vi "Actor Core.vi"(8 "error in":errorcluster, 11 "Jobber Proxy in":refnum<class "Jobber Proxy.lvclass">) -> (0 "error out":errorcluster, 3 "Actor out":refnum<class "Actor.lvclass">)   [LabVIEW 2014, in "Jobber Proxy.lvlib" / "Jobber Proxy.lvclass"]
doc: "(<B>Filename</B>: Actor Framework.lvlib:Actor.lvclass:Actor Core.vi)\n\nReceives messages to the actor, reacts to them, and initiates any error handling that may shut the actor down.\n\nDescendant classes may override this VI to append parallel tasks for the actor to complete while it handles messages. Overrides use the Call Parent Method node."
uses:
  Jobber Proxy.lvclass
  <vilib>/ActorFramework/Actor/Actor.lvclass
  Jobber/Jobber/Jobber.lvclass
  Jobber Proxy.lvclass/Jobber Proxy.ctl
  Jobber/Jobber/Jobber.lvclass/Jobber.ctl
  Classes/LabVIEW Instance/LabVIEW Instance.lvclass
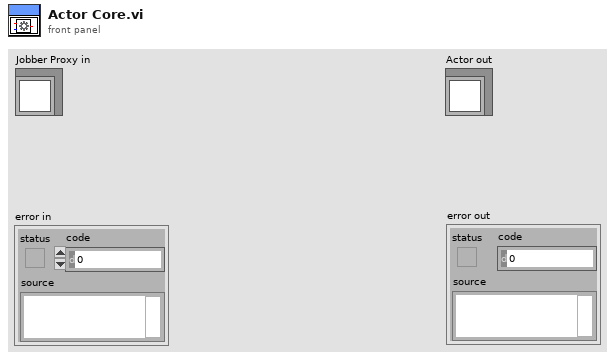
[diagram p1: front panel]
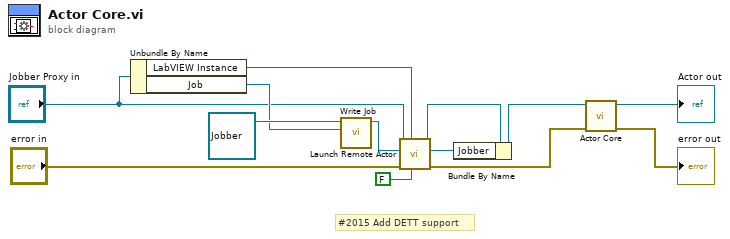
[diagram p0: block diagram]
diagram:
  # "#2015 Add DETT support"
  n1 = Unbundle By Name("Jobber Proxy in") -> ("LabVIEW Instance"=w6:refnum<class "LabVIEW Instance.lvclass">, "Job"=w7:refnum<class "Job.lvclass">)
  n2 = call "Write Job.vi"("Job.lvclass"=w7, "Jobber in"=refnum<class "Jobber.lvclass"> refnum ("Jobber.lvlib:Jobber.lvclass")) -> ("Jobber out"=w5:refnum<class "Jobber.lvclass">)  [unwired: 9 in]
  n3 = call "Launch Remote Actor.vi"("Open Actor Core front panel? (F)"=FALSE, "LabVIEW Instance in"=w6, "error in (no error)"="error in", "Nested Actor"=w5, "Caller Actor in"="Jobber Proxy in") -> ("error out"=w9:errorcluster, "Nested Actor's Enqueuer"=w4:refnum<class "Message Enqueuer.lvclass">, "Caller Actor out"=w3:refnum<class "Jobber Proxy.lvclass">)  [unwired: 4 in]
  n4 = Bundle By Name(cluster=w3, "Jobber"=w4) -> (w12:refnum<class "Jobber Proxy.lvclass">)
  n5 = call-parent "Actor Core.vi"("error in"=w9, "Actor in"=w12) -> ("error out"=→"error out":errorcluster, "Actor out"=→"Actor out":refnum<class "Actor.lvclass">)  [unwired: 8 in]
